vi "X sort-20220125.vi"(11 "x":dbl[](array[numeric])) -> (1 "Array 3":dbl[](array[numeric]), 2 "Array 2":dbl[](array[numeric]), 3 "Array":dbl[](array[numeric]), 4 "x > y?":bool[](array[boolean]), 5 "size(s)":i32)   [LabVIEW 2019]
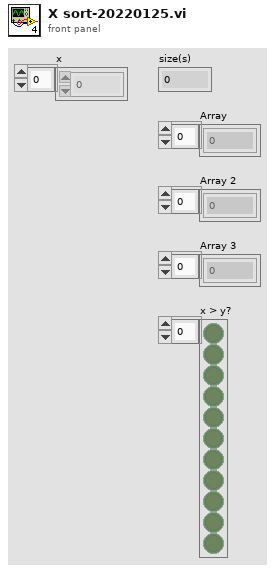
[diagram p1: front panel]
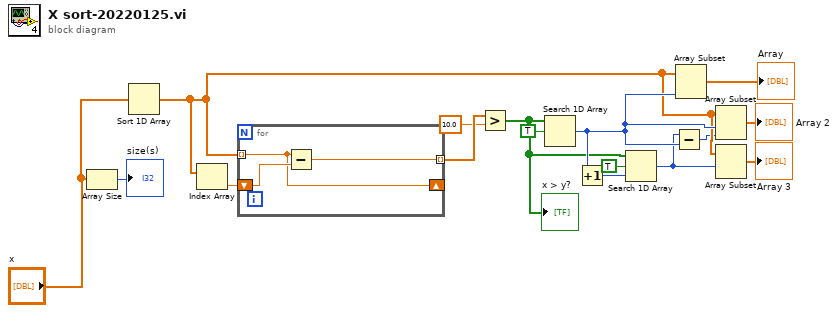
[diagram p0: block diagram]
diagram:
  n1 = Array Size(array="x") -> (size(s)=→"size(s)":i32)
  n2 = Sort 1D Array(array="x") -> (sorted array=w14:dbl[])
  n3 = Index Array(array=w14) -> (element=w1:dbl)  [unwired: 1 in]
  n4 = for {
    tunnel: w14 -> [w17] mode=indexing
    shift-right: [w17] -> _
    shift-left: w1 -> [w19]
    tunnel: [w18] -> w9 mode=indexing
    n5 = Subtract(x=w17, y=w19) -> (x-y=w18:dbl)
  }
  n6 = Greater?(x=w9, y=10.0) -> (0:w7:bool[])
  "x > y?" <- w7
  n7 = Search 1D Array(1D array=w7, element=TRUE) -> (index of element=w16:i32)  [unwired: 1 in]
  n8 = Increment(x=w16) -> (x+1=w15:i32)
  n9 = Search 1D Array(1D array=w7, element=TRUE, start index (0)=w15) -> (index of element=w10:i32)
  n10 = Subtract(x=w10, y=w16) -> (x-y=w8:i32)
  n11 = Array Subset(array=w14, length=w16) -> (→"Array":dbl[])  [unwired: 1 in]
  n12 = Array Subset(array=w14, index=w16, length=w8) -> (→"Array 2":dbl[])
  n13 = Array Subset(array=w14, index=w10) -> (→"Array 3":dbl[])  [unwired: 1 in]
